vi "Snap to Grid Position.vi"(10 "Gride Size (12px)":i32=12, 11 "Abs Position":i32) -> (3 "Resolved Abs Position":i32)   [LabVIEW 2019, in "Builtins.lvlib"]
doc: "Resolves the position to the nearest grid size. The grid size must be larger than 1.\n\nCreated by: Ryan Pacini"
uses:
  Builtins.lvlib
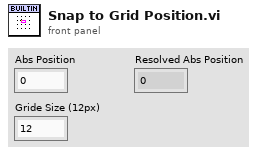
[diagram p1: front panel]
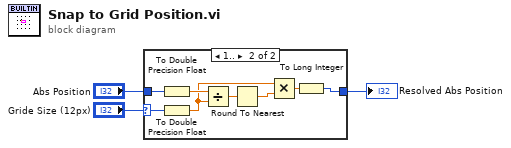
[diagram p0: block diagram]
diagram:
  n1 = case shown="1.." "Gride Size (12px)" {
    selector: "Gride Size (12px)" -> [_ w5]
    tunnel: "Abs Position" -> [w4 w9]
    tunnel: [w4 w6] -> w2
    frame ..0 {
      # "no difference"
    }
    frame 1.. {
      n2 = To Double Precision Float(number=w9) -> (double precision float=w11:dbl)
      n3 = To Double Precision Float(number=w5) -> (double precision float=w8:dbl)
      n4 = Divide(x=w11, y=w8) -> (x/y=w12:dbl)
      n5 = Round To Nearest(number=w12) -> (nearest integer value=w10:dbl)
      n6 = Multiply(x=w8, y=w10) -> (x*y=w7:dbl)
      n7 = To Long Integer(number=w7) -> (32bit integer=w6:i32)
    }
  }
  "Resolved Abs Position" <- w2
